vi "Configure Pulse Width Trigger.vi"(0 "VISA resource name":refnum<visa-resource-name>, 1 "Width":dbl=2e-05, 5 "Function":u16(ring) items=["Voltage: DC", "Voltage: AC", "Current: DC", "Current: AC", "2W Resistance", "4W Resistance", "Diode", "Capacitance", "Temperature", "Continuity", "Frequency", "Period", "Ratio", "Digitize Voltage", "Digitize Current"], 7 "Pulse Condition":u16(ring) items=["Greater", "Less"], 9 "Level":dbl, 11 "error in (no error)":errorcluster, 12 "HF Rejection":bool=TRUE) -> (4 "VISA resource name out":refnum<visa-resource-name>, 15 "error out":errorcluster)   [LabVIEW 2016, in "Keithley DMM7510.lvlib"]
doc: "This VI sets the slope and level of the analog edge trigger. This also enables or disables the high frequency rejection for analog trigger."
uses:
  Keithley DMM7510.lvlib
panel:
  in  "Polarity":u16(ring) items=["Above", "Below"]
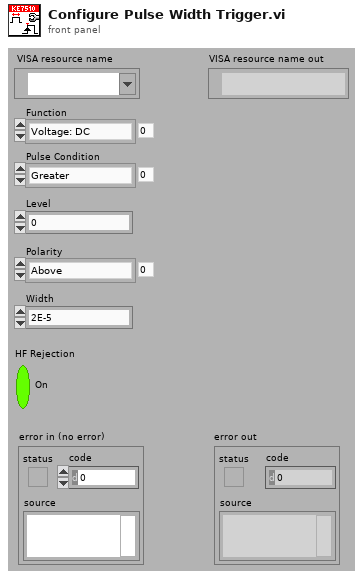
[diagram p1: front panel]
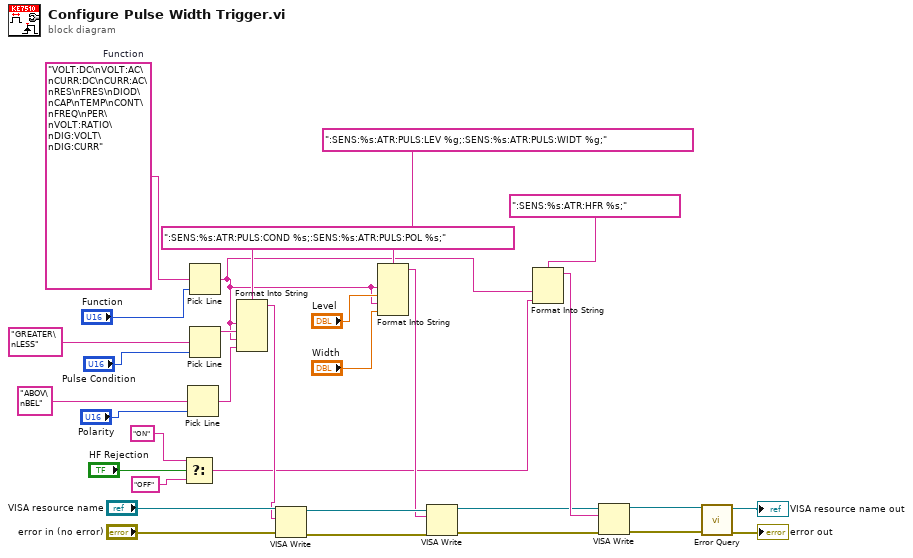
[diagram p0: block diagram]
diagram:
  w27 = "VOLT:DC\nVOLT:AC\nCURR:DC\nCURR:AC\nRES\nFRES\nDIOD\nCAP\nTEMP\nCONT\nFREQ\nPER\nVOLT:RATIO\nDIG:VOLT\nDIG:CURR"  # Function
  n1 = Select(t="ON" ("format string"), s="HF Rejection", f="OFF" ("format string")) -> (s? t:f=w7:string)
  n2 = Pick Line(multi-line string="ABOV\nBEL", line index="Polarity") -> (output string=w4:string)  [unwired: 1 in]
  n3 = Pick Line(multi-line string=w27, line index="Function") -> (output string=w3:string)  [unwired: 1 in]
  n4 = Pick Line(multi-line string="GREATER\nLESS", line index="Pulse Condition") -> (output string=w25:string)  [unwired: 1 in]
  n5 = Format Into String(format string=":SENS:%s:ATR:PULS:COND %s;:SENS:%s:ATR:PULS:POL %s;", w3, w25, w3, w4) -> (resulting string=w19:string)  [unwired: 2 in, 1 out]
  n6 = VISA Write(VISA resource name="VISA resource name", write buffer=w19, error in (no error)="error in (no error)") -> (VISA resource name out=w18:refnum<visa-resource-name>, error out=w17:errorcluster)  [unwired: 1 out]
  n7 = Format Into String(format string=":SENS:%s:ATR:PULS:LEV %g;:SENS:%s:ATR:PULS:WIDT %g;", w3, "Level", w3, "Width") -> (resulting string=w16:string)  [unwired: 2 in, 1 out]
  n8 = VISA Write(VISA resource name=w18, write buffer=w16, error in (no error)=w17) -> (VISA resource name out=w11:refnum<visa-resource-name>, error out=w8:errorcluster)  [unwired: 1 out]
  n9 = Format Into String(format string=":SENS:%s:ATR:HFR %s;", w3, w7) -> (resulting string=w12:string)  [unwired: 2 in, 1 out]
  n10 = VISA Write(VISA resource name=w11, write buffer=w12, error in (no error)=w8) -> (VISA resource name out=w10:refnum<visa-resource-name>, error out=w9:errorcluster)  [unwired: 1 out]
  n11 = call "Error Query.vi"("error in (no error)"=w9, "VISA resource name"=w10) -> ("error out"=→"error out":errorcluster, "VISA resource name out"=→"VISA resource name out":refnum<visa-resource-name>)  [unwired: 6 in, 2 out]
